vi "Calibrate Automatic Result.vi"(8 "error in":errorcluster, 11 "Instrument Handle In":i32) -> (0 "error out":errorcluster, 2 "Result":i32(ring) items=["Pass", "Fail, did not converge", "Corrupt"], 3 "Instrument Handle Out":i32)   [LabVIEW 8.6, in "ZTScopeM.lvlib"]
doc: "Queries the instrument to get the calibration result."
uses:
  ZTScopeM.lvlib
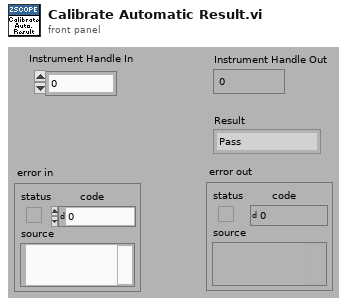
[diagram p1: front panel]
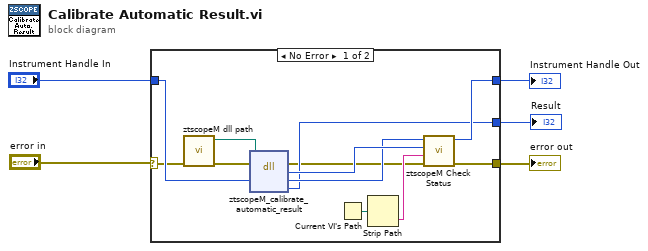
[diagram p0: block diagram]
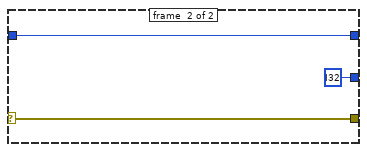
[diagram p2: hidden frame]
diagram:
  n1 = case shown="No Error" "error in" {
    selector: "error in" -> [w10 w20]
    tunnel: [w12 w20] -> w2
    tunnel: "Instrument Handle In" -> [w17 w19]
    tunnel: [w11 w19] -> w4
    tunnel: [w8 i32 ? ("Result")] -> w1
    frame #0 {
      n2 = call "ztscopeM dll path.vi"("error in (no error)"=w10) -> ("error out"=w7:errorcluster, "<instrument>.dll path"=w9:path)  [unwired: 9 in]
      n3 = dll-call lib="C:/Projects/codedepot/Teradyne/2016-1034 Teradyne ZScope API/Software/LabVIEW src/ztScopeM/Public/ztscopeM.dll" fn="ztscopeM_calibrate_automatic_result"(path in=w9, error in=w7, "instrumentHandle"=w17) -> (error out=w6:errorcluster, "return type"=w14:i32, "instrumentHandle"=w13:i32, "Result"=w8:i32)  [unwired: 2 in, 1 out]
      n4 = Current VI's Path() -> (path=w16:path)
      n5 = Strip Path(path=w16) -> (name=w15:string)  [unwired: 1 out]
      n6 = call "ztscopeM Check Status.vi"("error in"=w6, "name of VI"=w15, "status (return code)"=w14, "instrument handle in"=w13) -> ("error out"=w12:errorcluster, "instrument handle out"=w11:i32)  [unwired: 2 in]
    }
    frame #1 {
    }
  }
  "Instrument Handle Out" <- w4
  "error out" <- w2
  "Result" <- w1
